vi "handler_motor.vi"(8 "error in (no error)":errorcluster, 11 "HTTP Request in":T1) -> (0 "error out":errorcluster, 1 "Handler name":string, 3 "HTTP Request out":T1)   [LabVIEW 2011]
uses:
  template_field_type.ctl
  template_field.ctl
  http_request.ctl
  http_field.ctl
  http_response.ctl
  http_request_response.ctl
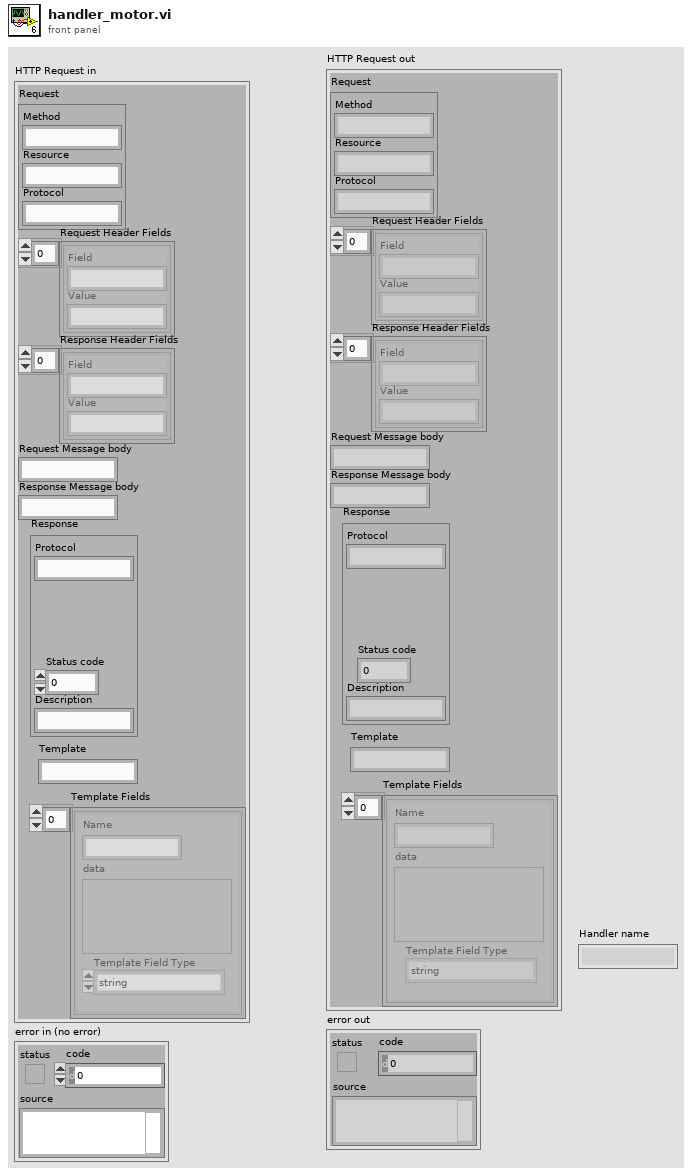
[diagram p1: front panel]
types:
  T1 = typedef "http_request_response.ctl" = cluster{"Request":T2, "Request Header Fields":T3[], "Response Header Fields":T3[], "Request Message body":string, "Response Message body":string, "Response":T4, "Template":string, "Template Fields":T5[]}
  T2 = typedef "http_request.ctl" = cluster{"Method":string, "Resource":string, "Protocol":string}
  T3 = typedef "http_field.ctl" = cluster{"Field":string, "Value":string}
  T4 = typedef "http_response.ctl" = cluster{"Protocol":string, "Status code":dbl, "Description":string}
  T5 = typedef "template_field.ctl" = cluster{"Name":string, "Template Field Type":T6, "data":variant}
  T6 = typedef "template_field_type.ctl" = enum16{"string", "string array", "number", "number array", "cluster", "cluster array"}
  T7 = typedef "html_form_field.ctl" = cluster{"field name":string, "field value":string}
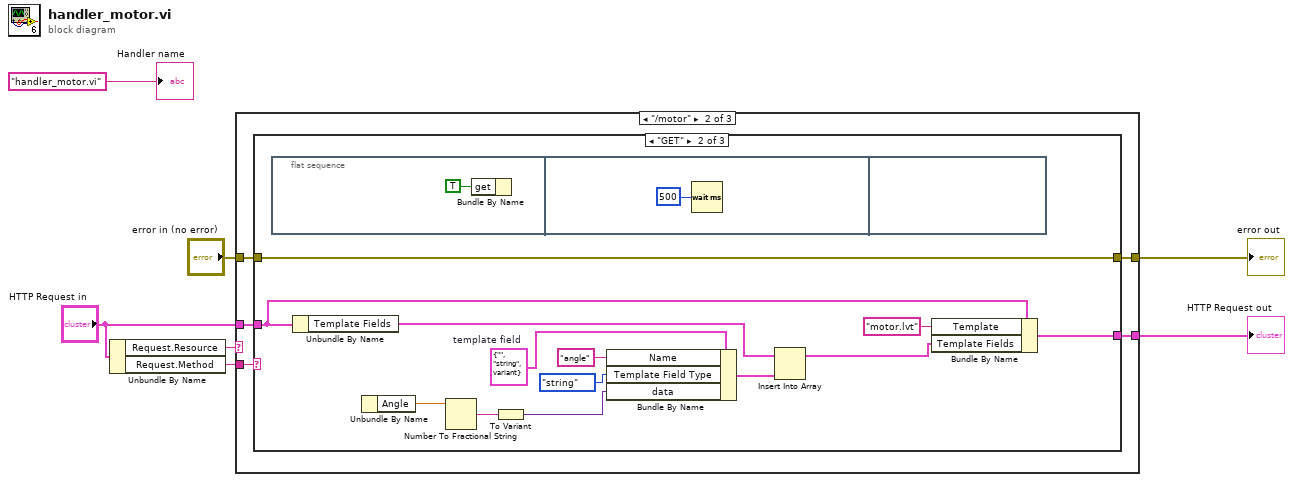
[diagram p0: block diagram]
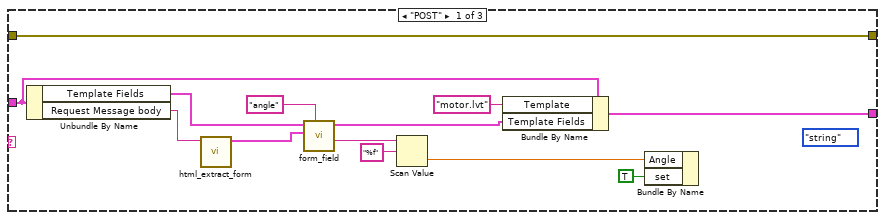
[diagram p3: hidden frame]
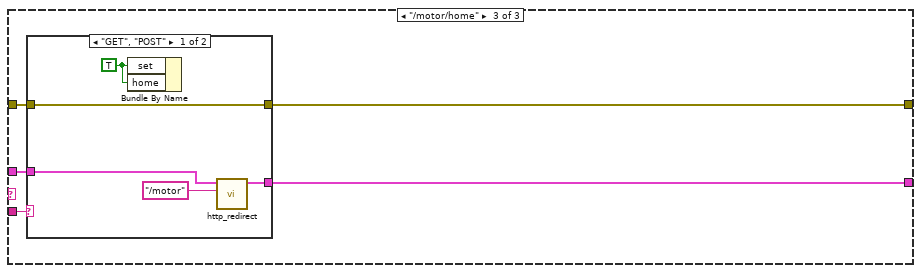
[diagram p5: hidden frame]
diagram:
  n1 = Unbundle By Name("HTTP Request in") -> ("Request.Resource"=w3:string, "Request.Method"=w2:string)
  n2 = case shown="\"/motor\"" w3 {
    tunnel: w2 -> [_ w14 w49]
    tunnel: "HTTP Request in" -> [w9 w13 w48]
    tunnel: [w9 w12 w47] -> w6
    tunnel: "error in (no error)" -> [w8 w11 w46]
    tunnel: [w8 w10 w45] -> w5
    frame Default {
    }
    frame "/motor" {
      n3 = case shown="\"GET\"" w14 {
        tunnel: w13 -> [w25 w32 w44]
        tunnel: [w26 w39 w44] -> w12
        tunnel: w11 -> [w27 w40 w43]
        tunnel: [w27 w40 w43] -> w10
        frame "POST" {
          (unwired) template_field_type."string" ("Template Field Type")
          n4 = Unbundle By Name(w25) -> ("Template Fields"=w17:T5[], "Request Message body"=w24:string)
          n5 = call "html_extract_form.vi"("Message Body"=w24) -> ("Form Data"=w18:T7[])  [unwired: 10 in]
          n6 = call "form_field.vi"("Name"="angle", "Form Data"=w18, "Template Fields"=w17) -> ("field value"=w15:string, "Template Fields"=w16:T5[])  [unwired: 6 in, 1 out]
          n7 = Scan Value(string=w15, format string="%f") -> (value=w21:dbl)  [unwired: 1 in, 1 out]
          n8 = Bundle By Name(cluster=w25, "Template"="motor.lvt", "Template Fields"=w16) -> (w26:T1)
          n9 = Bundle By Name("Angle"=w21, "set"=TRUE) -> ()  [unwired: 1 in, 1 out]
        }
        frame "GET" {
          w37 = T5 {"Name"="", "Template Field Type"=enum."string", "data"=variant}  # template field
          n10 = flat-sequence {
            frame #0 {
              n11 = Bundle By Name("get"=TRUE) -> ()  [unwired: 1 in, 1 out]
            }
            frame #1 {
              n12 = Wait (ms)(milliseconds to wait=u32 500) -> ()  [unwired: 1 out]
            }
            frame #2 {
            }
          }
          n13 = Unbundle By Name(w32) -> ("Template Fields"=w31:T5[])
          n14 = Unbundle By Name() -> ("Angle"=w29:dbl)  [unwired: 1 in]
          n15 = Number To Fractional String(number=w29) -> (F-format string=w28:string)  [unwired: 3 in]
          n16 = To Variant(anything=w28) -> (Variant=w34:variant)
          n17 = Bundle By Name(cluster=w37, "Name"="angle", "Template Field Type"=template_field_type."string", "data"=w34) -> (w36:T5)
          n18 = Insert Into Array(array=w31, new element=w36) -> (w30:T5[])  [unwired: 1 in]
          n19 = Bundle By Name(cluster=w32, "Template"="motor.lvt", "Template Fields"=w30) -> (w39:T1)
        }
        frame Default {
        }
      }
    }
    frame "/motor/home" {
      n20 = case shown="\"GET\", \"POST\"" w49 {
        tunnel: w48 -> [w52 w56]
        tunnel: [w53 w56] -> w47
        tunnel: w46 -> [w54 w55]
        tunnel: [w54 w55] -> w45
        frame "GET", "POST" {
          w50 = TRUE ("set")
          n21 = Bundle By Name("set"=w50, "home"=w50) -> ()  [unwired: 1 in, 1 out]
          n22 = call "http_redirect.vi"("Value"="/motor", "HTTP Request in in"=w52) -> ("HTTP Request in out"=w53:T1)  [unwired: 9 in]
        }
        frame Default {
        }
      }
    }
  }
  "HTTP Request out" <- w6
  "error out" <- w5
  "Handler name" <- "handler_motor.vi" ("Handler name")
